vi "SaveImageToFile.vi"(8 "error in (no error)":errorcluster, 10 "File Path":path, 11 "Image Pixels (U16)":u16[][](array[numeric])) -> (0 "error out":errorcluster)   [LabVIEW 2017]
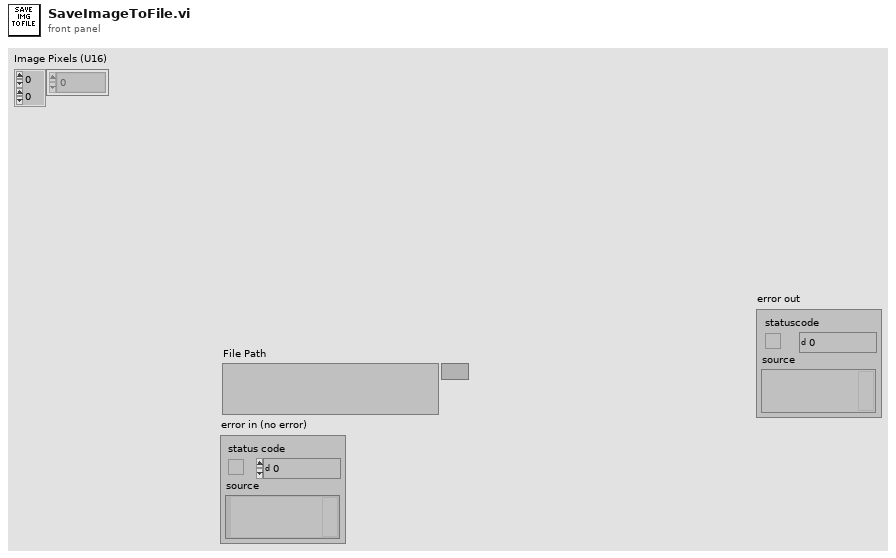
[diagram p1: front panel]
types:
  T1 = typedef "Image Type" = u32
  T2 = typedef "IMAQ Image.ctl" = refnum<image>
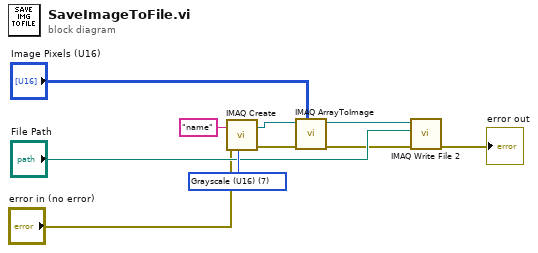
[diagram p0: block diagram]
diagram:
  w9 = T1 7 items=["Grayscale (U8)", "Grayscale (I16)", "Grayscale (SGL)", "Complex (CSG)", "RGB (U32)", "HSL (U32)", "RGB (U64)", "Grayscale (U16)"] ("Image Type")
  n1 = call "IMAQ Create"("Image Name"="name", "Image Type"=w9, "error in (no error)"="error in (no error)") -> ("New Image"=w3:T2, "error out"=w5:errorcluster)  [unwired: 2 in]
  n2 = call "IMAQ ArrayToImage"("Image Pixels (U16)"="Image Pixels (U16)", "error in (no error)"=w5, "Image"=w3) -> ("error out"=w4:errorcluster, "Image Out"=w8:T2)  [unwired: 7 in]
  n3 = call-poly "IMAQ Write File 2"("error in (no error)"=w4, "File Path"="File Path", "Image"=w8) -> ("error out"=→"error out":errorcluster)  [unwired: 7 in, 1 out]
